vi "P2.vi"() -> ()   [LabVIEW 2019]
panel:
  in  "#3":dbl
  in  "#2":dbl
  in  "#1":dbl
  out "(c)=(a)*(b)":dbl
  out "(b)Random Number":dbl
  out "(a)Average":dbl
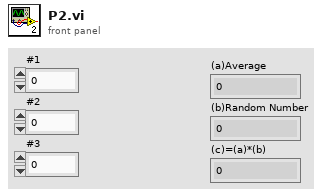
[diagram p1: front panel]
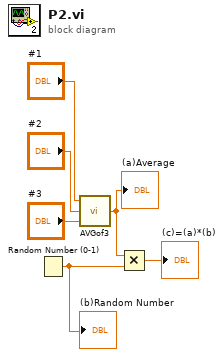
[diagram p0: block diagram]
diagram:
  n1 = Random Number (0-1)() -> (number: 0 to 1=w5:dbl)
  "(b)Random Number" <- w5
  n2 = call "AVGof3.vi"("Input c"="#3", "Input b"="#2", "Input a"="#1") -> ("Average of a,b,c"=w4:dbl)
  "(a)Average" <- w4
  n3 = Multiply(x=w4, y=w5) -> (x*y=→"(c)=(a)*(b)":dbl)
